vi "SSH_TUNNEL_Setup.vi"(0 "SSH_TUNNEL in":refnum<class "SSH_TUNNEL.lvclass">, 1 "ssh hostname":string, 2 "ssh host port":i32, 3 "username":string, 4 "password":string, 5 "error in (no error)":errorcluster) -> (14 "SSH_TUNNEL out":refnum<class "SSH_TUNNEL.lvclass">, 19 "error out":errorcluster)   [LabVIEW 2018, in "SSH_TUNNEL.lvclass"]
uses:
  SSH_TUNNEL.lvclass
  SSH_TUNNEL.lvclass/SSH_TUNNEL.ctl
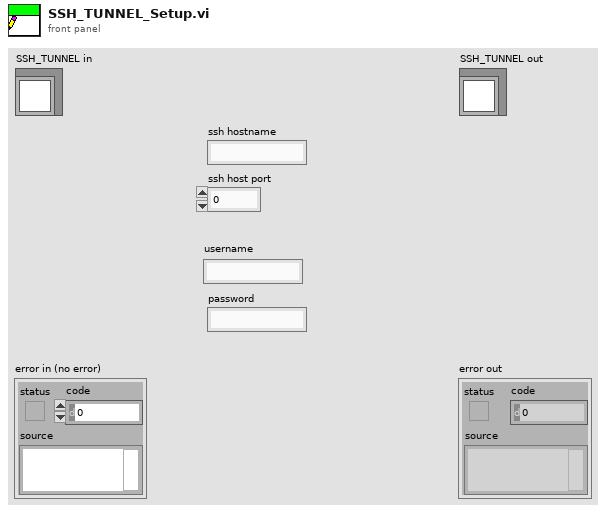
[diagram p1: front panel]
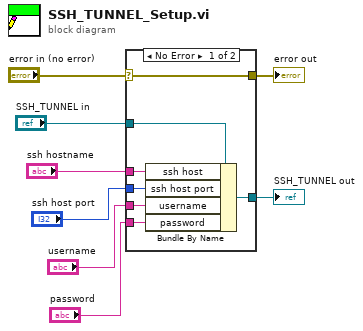
[diagram p0: block diagram]
diagram:
  n1 = case shown="No Error" "error in (no error)" {
    selector: "error in (no error)" -> [w15 w16]
    tunnel: [w15 w16] -> w7
    tunnel: [w13 w17] -> w5
    tunnel: "SSH_TUNNEL in" -> [w14 w17]
    tunnel: "ssh hostname" -> [w12 _]
    tunnel: "username" -> [w11 _]
    tunnel: "ssh host port" -> [w10 _]
    tunnel: "password" -> [w9 _]
    frame No Error {
      n2 = Bundle By Name(cluster=w14, "ssh host"=w12, "ssh host port"=w10, "username"=w11, "password"=w9) -> (w13:refnum<class "SSH_TUNNEL.lvclass">)
    }
    frame Error {
    }
  }
  "error out" <- w7
  "SSH_TUNNEL out" <- w5
